vi "ExQCircBufROI.vi"() -> ()   [LabVIEW 2010]
uses:
  Open-Close/CamHandle.vi
panel:
  in  "ADC Gain":u32
  out "ADC Speed (Khz)":u32
  in  "Fast ADC":bool
  in  "X Start":u32=1 min=1 step=1
  in  "Y Bin":u32=1 min=1 step=1
  in  "X End":u32=512 min=1 max=10000 step=1
  in  "X Bin":u32=1 min=1 step=1
  in  "Y Start":u32=1 min=1 step=1
  in  "Y End":u32=512 min=1 max=10000 step=1
  in  "Temperature":dbl format="%.2f"
  in  "Exposure":dbl min=0.0 step=0.001 format="%.3f"
  in  "stop":bool
  in  "Store":bool
  out "error out":errorcluster
  in  "error in (no error)":errorcluster
  # "ExQCircBufROI:\nThis example allows a single ROI\nto be programmed up. It then runs\nin sync (focus) mode displaying \nthe ROI data as it comes in.\nNote: this example requires the \ncamera support circular buffers."
  # "NOTICE\n\nTHIS VI USES A GLOBAL CAMERA HANDLE\n\nTHE VI EXOPENGLOBALCAM.VI MUST BE\nRUN AT THE START OF THE WORK SESSION.\nTHE CAMERA WILL REMAIN OPENED.\n\nTHE VI EXCLOSEGLOBALCAM.VI MUST\nBE RUN BEFORE LEAVING LABVIEW."
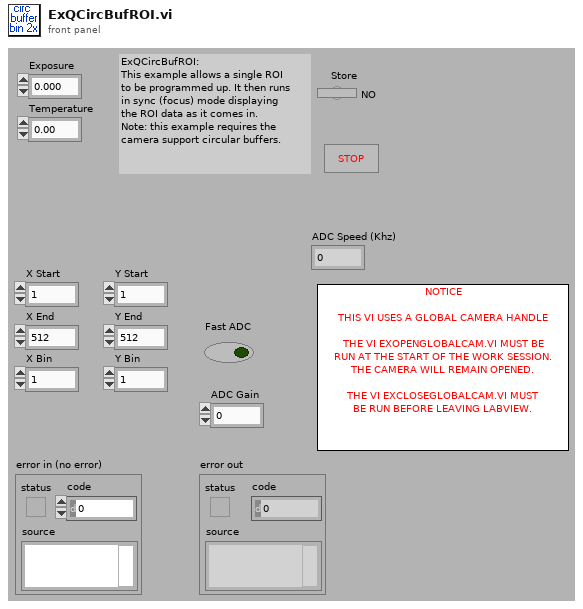
[diagram p1: front panel]
types:
  T1 = cluster{"X Start":u32, "X End":u32, "X Bin":u32, "Y Start":u32, "Y End":u32, "Y Bin":u32}
  T2 = cluster{"acquire focus mode":u32, "Exposure":dbl, "Number of Images":u32, "Software accumulation":u32}
  T3 = cluster{"Camera Handle":u32, "File Handle":u32, "Display Handle":u32, "Image Handle":u32}
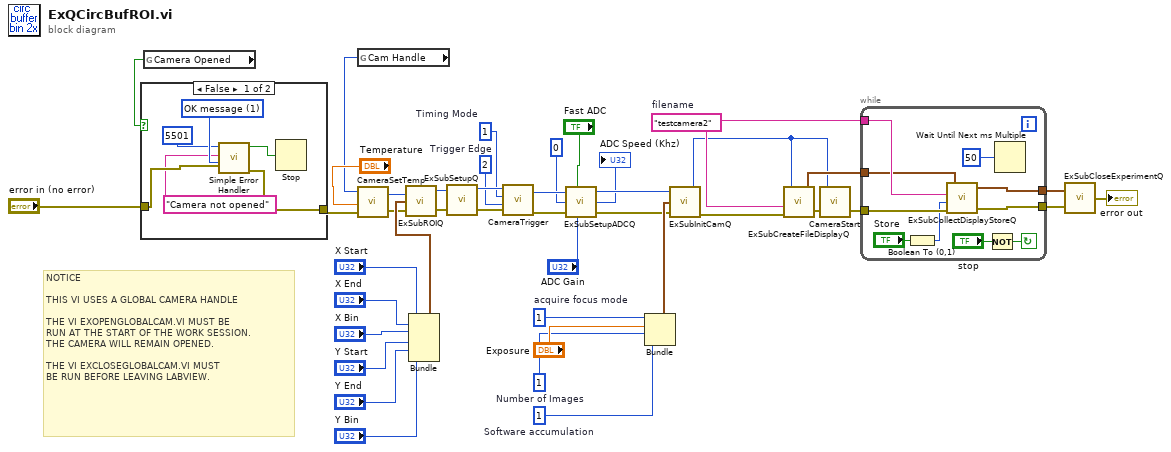
[diagram p0: block diagram]
diagram:
  w27 = u32 1  # Timing Mode
  w28 = u32 2  # Trigger Edge
  w31 = u32 1  # acquire focus mode
  w30 = u32 1  # Number of Images
  w29 = u32 1  # Software accumulation
  w42 = "testcamera2"  # filename
  # "NOTICE\n\nTHIS VI USES A GLOBAL CAMERA HANDLE\n\nTHE VI EXOPENGLOBALCAM.VI MUST BE\nRUN AT THE START OF THE WORK SESSION.\nTHE CAMERA WILL REMAIN OPENED.\n\nTHE VI EXCLOSEGLOBALCAM.VI MUST\nBE RUN BEFORE LEAVING LABVIEW."
  n1 = global read "CamHandle.vi" "Camera Opened"() -> (w2:bool)
  n2 = case shown="False" w2 {
    tunnel: "error in (no error)" -> [w47 w49]
    tunnel: [w46 w49] -> w3
    frame False {
      w48 = u16 1 items=["no dialog", "OK message", "continue or stop message"] ("type of dialog (OK msg:1)")
      n3 = call <vilib>:"Simple Error Handler.vi"("error code (no error:0)"=5501, "error source (\" \")"="Camera not opened", "type of dialog (OK msg:1)"=w48, "error in (no error)"=w47) -> ("error?"=w44:bool, "error out"=w46:errorcluster)  [unwired: 1 in, 3 out]
      n4 = Stop(stop? (T)=w44) -> ()
    }
    frame True {
    }
  }
  n5 = global read "CamHandle.vi" "Cam Handle"() -> (w1:u32)
  n6 = call <userlib>:"CameraSetTemp.vi"("error in (no error)"=w3, "Temperature"="Temperature", "Camera Handle"=w1) -> ("error out"=w17:errorcluster, "Camera Handle"=w16:u32)
  n7 = Bundle("X Start"="X Start", "X End"="X End", "X Bin"="X Bin", "Y Start"="Y Start", "Y End"="Y End", "Y Bin"="Y Bin") -> (w19:T1)  [unwired: 1 in]
  n8 = call "ExSubROIQ.vi"("error in (no error)"=w17, "ROI"=w19, "Camera Handle"=w16) -> ("error out"=w14:errorcluster, "Camera Handle"=w18:u32)
  n9 = call "ExSubSetupQ.vi"("error in (no error)"=w14, "Camera Handle"=w18) -> ("error out"=w13:errorcluster, "Camera Handle"=w34:u32)
  n10 = call <userlib>:"CameraTrigger.vi"("error in"=w13, "Trigger Edge"=w28, "Timing Mode"=w27, "Camera Handle"=w34) -> ("error out"=w11:errorcluster, "Camera Handle"=w12:u32)
  n11 = call "ExSubSetupADCQ.vi"("Camera Handle"=w12, "Fast ADC"="Fast ADC", "ReadOut Port"=0, "error in (no error)"=w11, "ADC Gain"="ADC Gain") -> ("Camera Handle"=w9:u32, "ADC Speed (Khz)"=→"ADC Speed (Khz)":u32, "error out"=w10:errorcluster)
  n12 = Bundle("acquire focus mode"=w31, "Exposure"="Exposure", "Number of Images"=w30, "Software accumulation"=w29) -> (w40:T2)  [unwired: 1 in]
  n13 = call "ExSubInitCamQ.vi"("error in (no error)"=w10, "Camera Information"=w40, "Camera Handle"=w9) -> ("error out"=w39:errorcluster, "Camera Handle"=w26:u32)
  n14 = call "ExSubCreateFileDisplayQ.vi"("error in (no error)"=w39, "File and Display Name"=w42, "Camera Handle"=w26) -> ("error out"=w32:errorcluster, "Handles Out"=w38:T3)  [unwired: 1 in]
  n15 = call <userlib>:"CameraStart.vi"("error in"=w32, "Camera Handle"=w26) -> ("error out"=w33:errorcluster)  [unwired: 1 out]
  n16 = while {
    tunnel: w38 -> [w50]
    tunnel: w33 -> [w58]
    tunnel: w42 -> [w51]
    tunnel: [w56] -> w36
    tunnel: [w57] -> w37
    stop <- w54 continue-if-true
    n17 = Boolean To (0,1)(Boolean="Store") -> (0, 1=w52:i16)
    n18 = call "ExSubCollectDisplayStoreQ.vi"("error in (no error)"=w58, "Store flag"=w52, "Display Title"=w51, "Handle Cluster"=w50) -> ("error out"=w56:errorcluster, "Handle Cluster Out"=w57:T3)  [unwired: 1 out]
    n19 = Not(x="stop") -> (.not. x?=w54:bool)
    n20 = Wait Until Next ms Multiple(millisecond multiple=u32 50) -> ()  [unwired: 1 out]
  }
  n21 = call "ExSubCloseExperimentQ.vi"("error in (no error)"=w36, "Handles In"=w37) -> ("error out"=→"error out":errorcluster)
